vi "Convert Array to BMI.vi"(1 "pBMI Data":u8[](array[numeric])) -> (0 "pBMI":T1)   [LabVIEW 2013, in "VRI.lvlib"]
doc: "This VI is used to convert an array of U32 to the BMI cluster. This is needed because the DLL function cannot return the cluster directly."
uses:
  VRI.lvlib
  _Type Defs/BITMAPINFO.ctl
  _Type Defs/BITMAPINFOHEADER.ctl
  _Type Defs/RGBQUAD.ctl
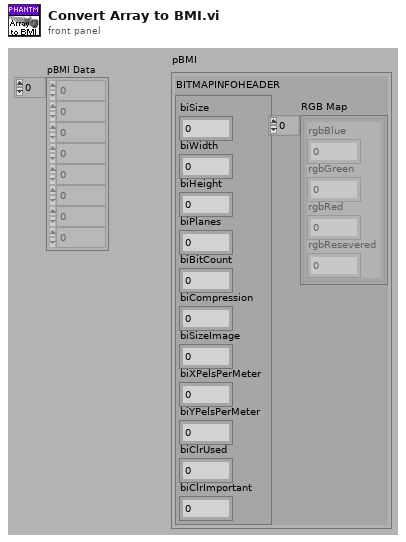
[diagram p1: front panel]
types:
  T1 = typedef "VRI.lvlib/BITMAPINFO.ctl" = cluster{"BITMAPINFOHEADER":T2, "RGB Map":T3[]}
  T2 = typedef "VRI.lvlib/BITMAPINFOHEADER.ctl" = cluster{"biSize":u32, "biWidth":i32, "biHeight":i32, "biPlanes":u16, "biBitCount":u16, "biCompression":u32, "biSizeImage":u32, "biXPelsPerMeter":i32, "biYPelsPerMeter":i32, "biClrUsed":u32, "biClrImportant":u32}
  T3 = typedef "VRI.lvlib/RGBQUAD.ctl" = cluster{"rgbBlue":u8, "rgbGreen":u8, "rgbRed":u8, "rgbResevered":u8}
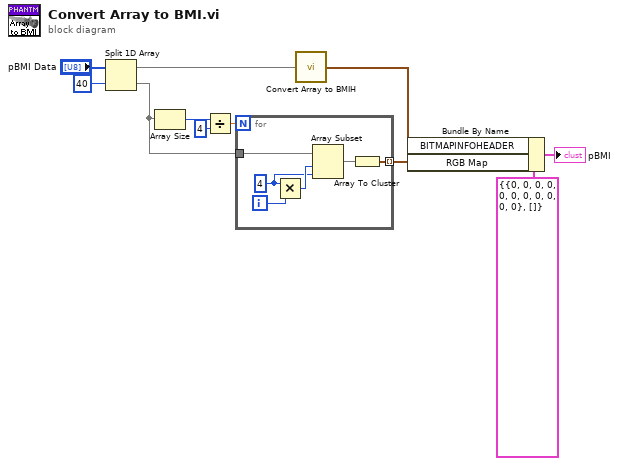
[diagram p0: block diagram]
diagram:
  n1 = Split 1D Array(array="pBMI Data", index=40 ("length")) -> (first subarray=w3:u8[], second subarray=w1:u8[])
  n2 = Array Size(array=w1) -> (size(s)=w7:i32)
  n3 = Divide(x=w7, y=4) -> (x/y=w6:dbl)
  n4 = for {
    N: w6 -> [_]
    tunnel: w1 -> [w15]
    tunnel: [w17] -> w4 mode=indexing
    i -> [w16]
    w13 = 4 ("x")
    n5 = Multiply(x=w13, y=w16) -> (x*y=w14:i32)
    n6 = Array Subset(array=w15, index=w14, length=w13) -> (w12:u8[])
    n7 = Array To Cluster(array=w12) -> (cluster=w17:cluster{"[0]":u8, "[1]":u8, "[2]":u8, "[3]":u8})
  }
  n8 = call "Convert Array to BMIH.vi"("Array"=w3) -> ("BITMAPINFOHEADER"=w2:T2)
  n9 = Bundle By Name(cluster=T1 {"BITMAPINFOHEADER"={"biSize"=0, "biWidth"=0, "biHeight"=0, "biPlanes"=0, "biBitCount"=0, "biCompression"=0, "biSizeImage"=0, "biXPelsPerMeter"=0, "biYPelsPerMeter"=0, "biClrUsed"=0, "biClrImportant"=0}, "RGB Map"=[]} ("pBMI 2"), "BITMAPINFOHEADER"=w2, "RGB Map"=w4) -> (→"pBMI":T1)
